vi "FTW-JSON-Array-Deserialize.vi"(5 "Array of JSON Objects":string, 11 "error in":errorcluster) -> (6 "JSON Elements":string[](array[string]), 8 "Valid Structure":bool, 15 "error out":errorcluster)   [LabVIEW 2015]
panel:
  # "Inputs"
  # "Outputs"
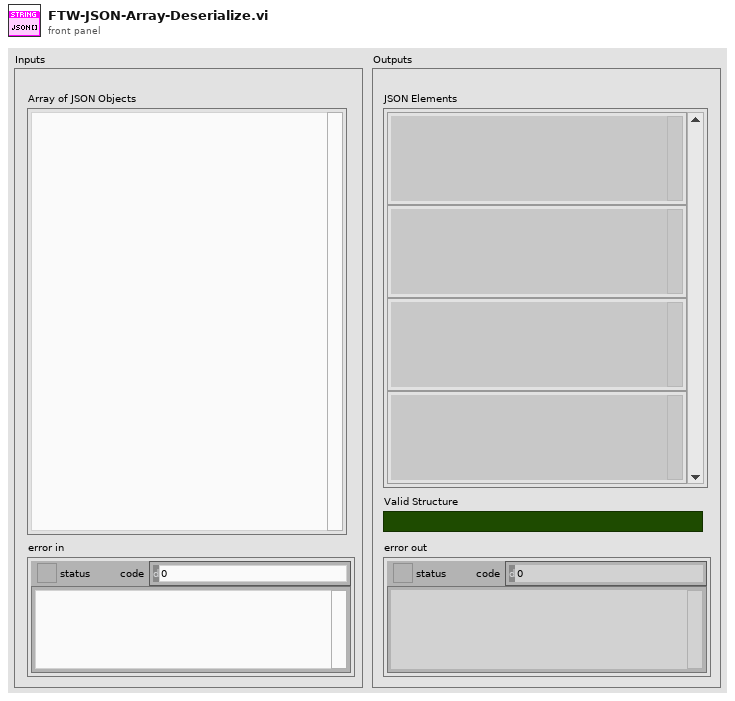
[diagram p1: front panel]
types:
  T1 = typedef "FTW-Type-JSON.ctl" = refnum<data-value>
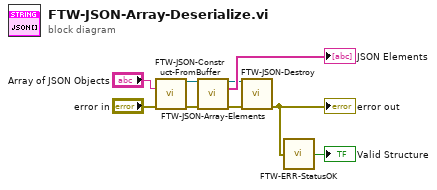
[diagram p0: block diagram]
diagram:
  n1 = call "FTW-JSON-Construct-FromBuffer.vi"("JSON String (UTF-8)"="Array of JSON Objects", "error in"="error in") -> ("JSON"=w3:T1, "error out"=w4:errorcluster)  [unwired: 12 in]
  n2 = call "FTW-JSON-Array-Elements.vi"("JSON"=w3, "error in"=w4) -> ("JSON out"=w1:T1, "Elements"=→"JSON Elements":string[], "error out"=w2:errorcluster)  [unwired: 11 in]
  n3 = call "FTW-JSON-Destroy.vi"("JSON"=w1, "error in"=w2) -> ("error out"=w9:errorcluster)  [unwired: 13 in]
  "error out" <- w9
  n4 = call "FTW-ERR-StatusOK.vi"("error to check"=w9) -> ("Status OK?"=→"Valid Structure":bool)
